vi "SeCrTs-Drive_Message.vi"(9 "Input":dbl, 11 "Packet \nIdentifier":i32=17) -> (2 "String":string)   [LabVIEW 2022 SP3]
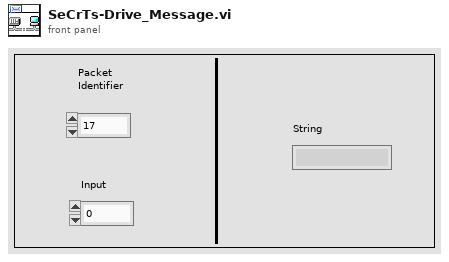
[diagram p1: front panel]
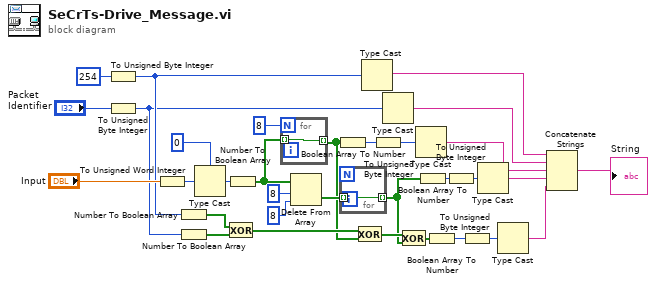
[diagram p0: block diagram]
diagram:
  n1 = To Unsigned Byte Integer(number=254) -> (unsigned 8bit integer=w11:u8)
  n2 = To Unsigned Byte Integer(number="Packet \nIdentifier") -> (unsigned 8bit integer=w10:u8)
  n3 = To Unsigned Word Integer(number="Input") -> (unsigned 16bit integer=w9:u16)
  n4 = Number To Boolean Array(number=w11) -> (Boolean array=w13:bool[])
  n5 = Number To Boolean Array(number=w10) -> (Boolean array=w12:bool[])
  n6 = Type Cast(type=i16 0, x=w9) -> (*(type *) &x=w26:i16)
  n7 = Exclusive Or(1:w12, 2:w13) -> (0:w4:bool[])
  n8 = Number To Boolean Array(number=w26) -> (Boolean array=w17:bool[])
  n9 = for {
    N: 8 -> [_]
    tunnel: w17 -> [w33] mode=indexing
    tunnel: [w33] -> w2 mode=indexing
  }
  n10 = Delete From Array(array=w17, length=8, index=8) -> (deleted portion=w20:bool[])  [unwired: 1 out]
  n11 = Boolean Array To Number(Boolean array=w2) -> (number=w22:u32)
  n12 = for {
    tunnel: w20 -> [w34] mode=indexing
    tunnel: [w34] -> w1 mode=indexing
  }
  n13 = Exclusive Or(1:w2, 2:w4) -> (0:w5:bool[])
  n14 = Type Cast(x=w11) -> (*(type *) &x=w29:string)  [unwired: 1 in]
  n15 = To Unsigned Byte Integer(number=w22) -> (unsigned 8bit integer=w23:u8)
  n16 = Type Cast(x=w10) -> (*(type *) &x=w28:string)  [unwired: 1 in]
  n17 = Exclusive Or(1:w1, 2:w5) -> (0:w6:bool[])
  n18 = Type Cast(x=w23) -> (*(type *) &x=w21:string)  [unwired: 1 in]
  n19 = Boolean Array To Number(Boolean array=w1) -> (number=w15:u32)
  n20 = Boolean Array To Number(Boolean array=w6) -> (number=w7:u32)
  n21 = To Unsigned Byte Integer(number=w15) -> (unsigned 8bit integer=w16:u8)
  n22 = To Unsigned Byte Integer(number=w7) -> (unsigned 8bit integer=w8:u8)
  n23 = Type Cast(x=w16) -> (*(type *) &x=w14:string)  [unwired: 1 in]
  n24 = Type Cast(x=w8) -> (*(type *) &x=w3:string)  [unwired: 1 in]
  n25 = Concatenate Strings(w29, w28, w21, w14, w3) -> (→"String":string)
